vi "Time.vi"(1 "Indice":dbl) -> (0 "Temps (s)":dbl)   [LabVIEW 2022 SP3]
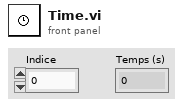
[diagram p1: front panel]
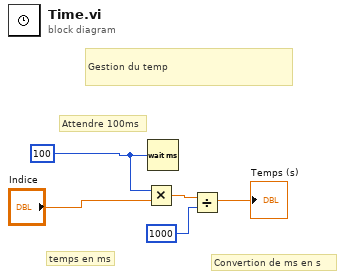
[diagram p0: block diagram]
diagram:
  w5 = u32 100 ("milliseconds to wait")
  # "temps en ms"
  # "Gestion du temp"
  # "Convertion de ms en s"
  # "Attendre 100ms"
  n1 = Multiply(x=w5, y="Indice") -> (x*y=w4:dbl)
  n2 = Wait (ms)(milliseconds to wait=w5) -> ()  [unwired: 1 out]
  n3 = Divide(x=w4, y=u32 1000) -> (x/y=→"Temps (s)":dbl)
